vi "Msg.Noti.Release.vi"(8 "Error (in)":errorcluster, 11 "Msg.Noti.Ref":T1) -> (0 "Error (out)":errorcluster)   [LabVIEW 2023]
uses:
  Msg.Noti.Ref.ctl
  Msg.Data.ctl
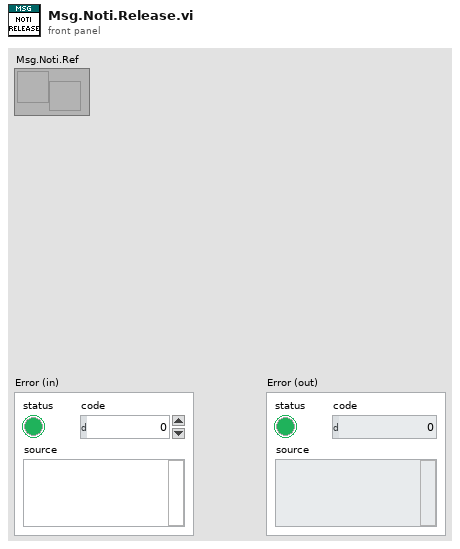
[diagram p1: front panel]
types:
  T1 = typedef "Msg.Noti.Ref.ctl" = refnum<notifier>
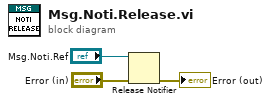
[diagram p0: block diagram]
diagram:
  n1 = Release Notifier(notifier="Msg.Noti.Ref", error in (no error)="Error (in)") -> (error out=→"Error (out)":errorcluster)  [unwired: 1 in, 2 out]
